vi "Main_v3.1.vi"() -> ()   [LabVIEW 2018]
doc: "Main VI for the controls"
uses:
  Components/PMCL Dynamic Signal Analyzer/Controls/DSA excitation specs.ctl
  Typedefs/StateDef_Enum.ctl
  <vilib>/Simulation/Scripting/Companion Diagram/SimConfigNode/SimParams.ctl
  <vilib>/Simulation/Scripting/Companion Diagram/SimConfigNode/_simSolvers.ctl
  <vilib>/Simulation/Implementation/Shared/SIMSCR Execution Mode.ctl
  <vilib>/Platform/TimedLoop/XDataNode/timing_clust.ctl
  <vilib>/Platform/TimedLoop/XDataNode/nitl_modes.ctl
  <vilib>/Platform/TimedLoop/XDataNode/wakeup.ctl
  <vilib>/Simulation/Param Hierarchy/Typedefs/SIMPH Param Control Actions.ctl
  <vilib>/Simulation/Implementation/Shared/SIM limit type.ctl
  <vilib>/Simulation/Scripting/Editor Utilities/SIM subVI tag data.ctl
  <vilib>/Simulation/Scripting/Editor Utilities/SIM subVI execution type.ctl
  <vilib>/Simulation/Implementation/Shared/NILVSim_ParamChanged.vi
  <vilib>/Simulation/Implementation/Shared/NILVSim_FinishedLate.vi
  <vilib>/Simulation/Implementation/Shared/NILVSIM_BeginStep.vi
  <vilib>/myRIO/Instrument Drivers/Onboard IO/AI/vis/Read.vi
  <vilib>/Simulation/Utility/Implementation/SIM SimulationParams.vi
  <vilib>/Simulation/ContinuousLinear/Implementation/NILVSim Integrator new.llb/SIM Integrator distributor (scalar).vi
  <vilib>/Simulation/Implementation/Shared/SIM Fire Discrete SubVI.vi
  <vilib>/Simulation/ContinuousLinear/Implementation/NILVSim Transfer Function Direct.llb/SIM Transfer Function Direct (SISO).vi
  <vilib>/Simulation/Utility/Implementation/SIM Halt.vi
  <vilib>/Simulation/SignalArithmetic/Implementation/NILVSim Gain.llb/SIM Gain (scalar).vi
  <vilib>/Simulation/ContinuousLinear/Implementation/NILVSim Integrator new.llb/SIM Integrator collector (scalar).vi
  <vilib>/Simulation/Implementation/Shared/NILVSim_Manager.vi
  <vilib>/Utility/error.llb/Clear Errors.vi
  <vilib>/Simulation/Implementation/Shared/NILVSim_FinalizeModel.vi
  <vilib>/Simulation/Utility/Implementation/NILVSim SimulationParams (core).vi
  <vilib>/Simulation/Implementation/Shared/SIM Fire Discrete SubVI (Core).vi
  <vilib>/myRIO/Common/Instrument Driver Framework/myRIO v1.0/AI/vis/myRIO v1.0 Close AI.vi
  <vilib>/myRIO/Common/Instrument Driver Framework/myRIO v1.0/AO/vis/myRIO v1.0 Close AO.vi
  <vilib>/myRIO/Common/Instrument Driver Framework/myRIO v1.0/AI/vis/myRIO v1.0 Unreserve AI.vi
  <vilib>/myRIO/Common/Instrument Driver Framework/myRIO v1.0/AO/vis/myRIO v1.0 Unreserve AO.vi
  <vilib>/myRIO/Common/Instrument Driver Framework/myRIO v1.0/Resource Manager/vis/myRIO v1.0 Unreserve Channel List.vi
  <vilib>/myRIO/Common/Instrument Driver Framework/myRIO v1.0/AI/vis/myRIO v1.0 Build MUX Configuration AI.vi
  <vilib>/myRIO/Common/Instrument Driver Framework/myRIO v1.0/AO/vis/myRIO v1.0 Build MUX Configuration AO.vi
  <vilib>/myRIO/Common/Instrument Driver Framework/myRIO v1.0/Resource Manager/vis/myRIO v1.0 Unreserve Channel.vi
  <vilib>/myRIO/Common/Instrument Driver Framework/myRIO v1.0/Resource Manager/vis/myRIO v1.0 Build Mutex Name.vi
  <vilib>/Simulation/Implementation/Shared/SIM Unbundle Sim Info.vi
  <vilib>/Simulation/Implementation/Shared/SIMSH Read Queue.vi
  <vilib>/Simulation/Implementation/Shared/NILVSim_Initialize.vi
  <vilib>/Utility/error.llb/Error Cluster From Error Code.vi
  <vilib>/myRIO/Common/Instrument Driver Framework/myRIO v1.0/AI/vis/myRIO v1.0 Read AI.vi
  <vilib>/myRIO/Common/Instrument Driver Framework/myRIO v1.0/AO/vis/myRIO v1.0 Write AO.vi
  <vilib>/Simulation/Utility/Implementation/NILVSim Get Time and IsAcceptedStep.vi
  <vilib>/Simulation/Implementation/Shared/NILVSim_GetModelError.vi
  <vilib>/Simulation/Implementation/Shared/SIM Bundle Sim Info.vi
  <vilib>/myRIO/Common/Instrument Driver Framework/Utilities/vis/Configuration Manager.vi
  <vilib>/myRIO/Common/Instrument Driver Framework/Utilities/vis/IO Manager.vi
  <vilib>/myRIO/Common/Instrument Driver Framework/myRIO v1.0/myRIO v1.0 Close.vi
  <vilib>/Simulation/Scripting/Companion Diagram/SimConfigNode/SimDog.xnode
  <vilib>/Platform/TimedLoop/XDataNode/XDataNode.xnode
  <vilib>/Simulation/Implementation/XNodeFramework/SimXNode/SimX.xnode
  Components/Timing/Timing.lvlib
  <vilib>/myRIO/Instrument Drivers/Onboard IO/AI/AI.lvlib
  <vilib>/myRIO/Instrument Drivers/Onboard IO/AO/AO.lvlib
  <vilib>/Platform/TimedLoop/XDataNode/XDNodeRunTimeDep.lvlib
  <vilib>/Analysis/NI_AALPro.lvlib
  <vilib>/ptbypt/NI_PtbyPt.lvlib
  <vilib>/Simulation/ContinuousLinear/Implementation/NILVSim Integrator new.llb/SIM Integrator (scalar).vi
  <vilib>/Simulation/Implementation/Shared/NI_SIM_Implementation.lvlib
panel:
  in  "System Stop Button":bool
  in  "Pause chart?":bool
  in  "Controller Params":enum32{"Page 1"}(tab)
  in  "Kp":dbl=1.0 min=0.0
  in  "Controller On?":bool
  out "Status":string
  in  "Ref. Gen.":enum32{"Analog In", "Manual", "Wave Gen", "DSA"}(tab)=enum."Manual"
  in  "Ref. cmd.":dbl(slide) step=1.0 scale=-10.0..10.0 scale format="%#.1f"
  in  "Signal Cluster":T1={"phase"=0.0, "amplitude"=1.0, "frequency"=1.0, "offset"=1.0, "Signal"=enum."Square"} {"offset" format="%0.2f"; "frequency" format="%0.2f"; "amplitude" format="%0.2f"; "phase" format="%0.2f"}
  out "DSA \nRunning?":bool
  in  "Stop DSA":bool
  in  "Start DSA":bool
  in  "DSA excitation specs":T2={"Initial Freq. [Hz]"=10.0, "Final Freq. [Hz]"=999.0, "# pts. in interval"=50, "Samping Time [s]"=0.001, "Amplitude [V]"=10.0, "Offset [V]"=0.0, "Freq Units (F: rad/s, T: Hz)"=TRUE}
  in  "Loop Timing":enum32{"CD&Sim", "Ref. gen", "UI"}(tab)
  out "# Finished\nLate counter":dbl
  in  "CD&Sim\nLoop Rate (Hz)":dbl=2000.0 format="%#_4p"
  out "# Finished\nLate counter":dbl
  in  "Ref. Gen.\nLoop Rate (Hz)":dbl=2000.0 format="%#_4p"
  in  "UI Loop rate (Hz)":dbl=1000.0 format="%#_6p"
  in  "Display Waveforms":enum32{"Controller Signals", "DSA "}(tab)
  out "Control Effort":dbl(graph)
  out "Waveform Chart":cluster{"Double":dbl, "Numeric":dbl}(graph)
  out "Phase Bode Plot":cluster{dbl[], dbl[]}(graph)
  out "Magnitude Bode Plot":cluster{dbl[], dbl[]}(graph)
  out "DSA Signals":cluster{"Double":dbl, "Double":dbl}(graph)
  # "Connect the Reference Signal \nto C/AI 1 of the myRIO."
  # "Pinout Config.:\nPort C/AI0 : Plant output being read by the myRIO\nPort C/AI1 : Reference signal for the control loop\nPort C/AO0 : Control effort signal to the plant"
  # "Ensure the excitation specs, cycle specs and\nCH0, CH1 inputs to the droppable DSA in the\nDSA loop are correctly set before starting DSA."
  # "Control Loop Timing"
  # "Ref.  Gen. Loop Timing"
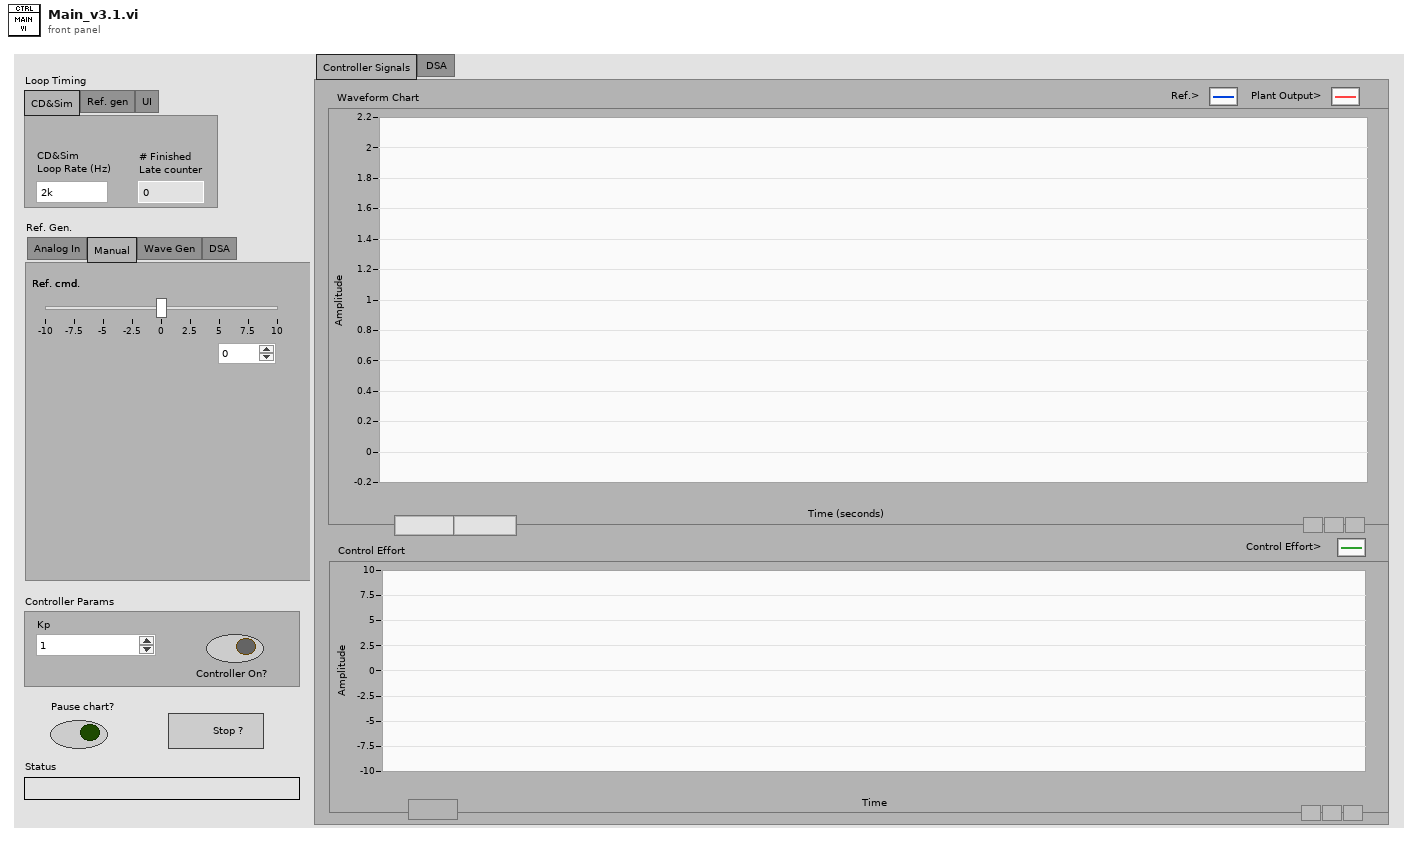
[diagram p1: front panel]
types:
  T1 = cluster{"phase":dbl, "amplitude":dbl, "frequency":dbl, "offset":dbl, "Signal":enum16{"Sine", "Square", "Sawtooth"}}
  T2 = typedef "DSA excitation specs.ctl" = cluster{"Initial Freq. [Hz]":dbl, "Final Freq. [Hz]":dbl, "# pts. in interval":i16, "Samping Time [s]":dbl, "Amplitude [V]":dbl, "Offset [V]":dbl, "Freq Units (F: rad/s, T: Hz)":bool}
  T3 = typedef "StateDef_Enum.ctl" = enum16{"Initialize", "Wait", "Shutdown"}
  T4 = typedef "XDNodeRunTimeDep.lvlib/timing_clust.ctl" = cluster{"Expected End [f-1]":u64, "Actual End [f-1]":u64, "Finished Late? [f-1]":bool, "Expected End [i-1]":u64, "Actual End [i-1]":u64, "Finished Late? [i-1]":bool, "Expected Start [i]":u64, "Actual Start [i]":u64, "Expected Start [f]":u64, "Actual Start [f]":u64, "Source Name":string, "Structure Name":string, "Period":i64, "Deadline":i64, "Offset":i64, "Start":i64, "Priority":i32, "Timeout":i32, "Mode":T5, "Wakeup Reason":T6, "Error":errorcluster, "Source Type":string, "Secondary Source Type":string, "Global End Time":u64, "Global Start Time":u64, "Frame Duration":u64, "Iteration Duration":u64, "Assigned CPU":i32, "I/O Scan Engine Mode":u32}
  T5 = typedef "XDNodeRunTimeDep.lvlib/nitl_modes.ctl" = enum32{"No Change", "Process missed periods, maintain original phase", "Discard missed periods, maintain original phase", "Process missed periods, ignore original phase", "Discard missed periods, ignore original phase"}
  T6 = typedef "XDNodeRunTimeDep.lvlib/wakeup.ctl" = enum32{"Normal", "Aborted", "Asynchronous wakeup", "Timing source error", "Timed loop error", "Timeout"}
  T7 = typedef "AI.lvlib/AI Reference.ctl" = cluster{"myRIO Reference":T8, "AI Channels List":T12, "AI Scaling Constants List":T14}
  T8 = typedef "myRIO Generic Hardware Reference.ctl" = cluster{"myRIO Model":T9, "myRIO Hardware Reference":T10}
  T9 = typedef "Hardware Version Enum.ctl" = enum16{"Unknown", "myRIO-1900", "myRIO-1950", "roboRIO", "NI ELVIS RIO CM", "ELVIS III"}
  T10 = typedef "myRIO v1.0 Reference.ctl" = cluster{"Generic FPGA Reference":T11, "Allow multiple opens":bool}
  T11 = typedef "Generic FPGA Reference.ctl" = refnum<k20>
  T12 = typedef "AI Channels List.ctl" = T13[]
  T13 = typedef "AI Channels Enum.ctl" = enum16{"Not Connected", "AudioIn/Left", "AudioIn/Right", "C/AI0", "C/AI1", "A/AI0", "A/AI1", "A/AI2", "A/AI3", "A/AI4", "A/AI5", "A/AI6", "A/AI7", "B/AI0", "B/AI1", "B/AI2", "B/AI3", "B/AI4", "B/AI5", "B/AI6", "B/AI7", "AI/AI0", "AI/AI1", "AI/AI2", "AI/AI3", "A/AI0 (DIFF)", "A/AI1 (DIFF)", "A/AI2 (DIFF)", "A/AI3 (DIFF)", "B/AI0 (DIFF)", "B/AI1 (DIFF)", "B/AI2 (DIFF)", "B/AI3 (DIFF)"}
  T14 = typedef "Analog Scaling Constants List.ctl" = T15[]
  T15 = typedef "Analog Scaling Constants.ctl" = cluster{"LSB Weight (Volts)":dbl, "Offset (Volts)":dbl, "Signed?":bool}
  T16 = typedef "AO.lvlib/AO Reference.ctl" = cluster{"myRIO Reference":T8, "AO Channel List":T17, "AO Scaling Constant List":T14}
  T17 = typedef "AO Channels List.ctl" = T18[]
  T18 = typedef "AO Channels Enum.ctl" = enum16{"Not Connected", "AudioOut/Left", "AudioOut/Right", "C/AO0", "C/AO1", "A/AO0", "A/AO1", "B/AO0", "B/AO1"}
  T19 = cluster{"Cycles To Settle (M)":i16, "Cycles To Calculate (N)":i16}
  T20 = cluster{"Analog In CH1":dbl, "Analog In CH0":dbl}
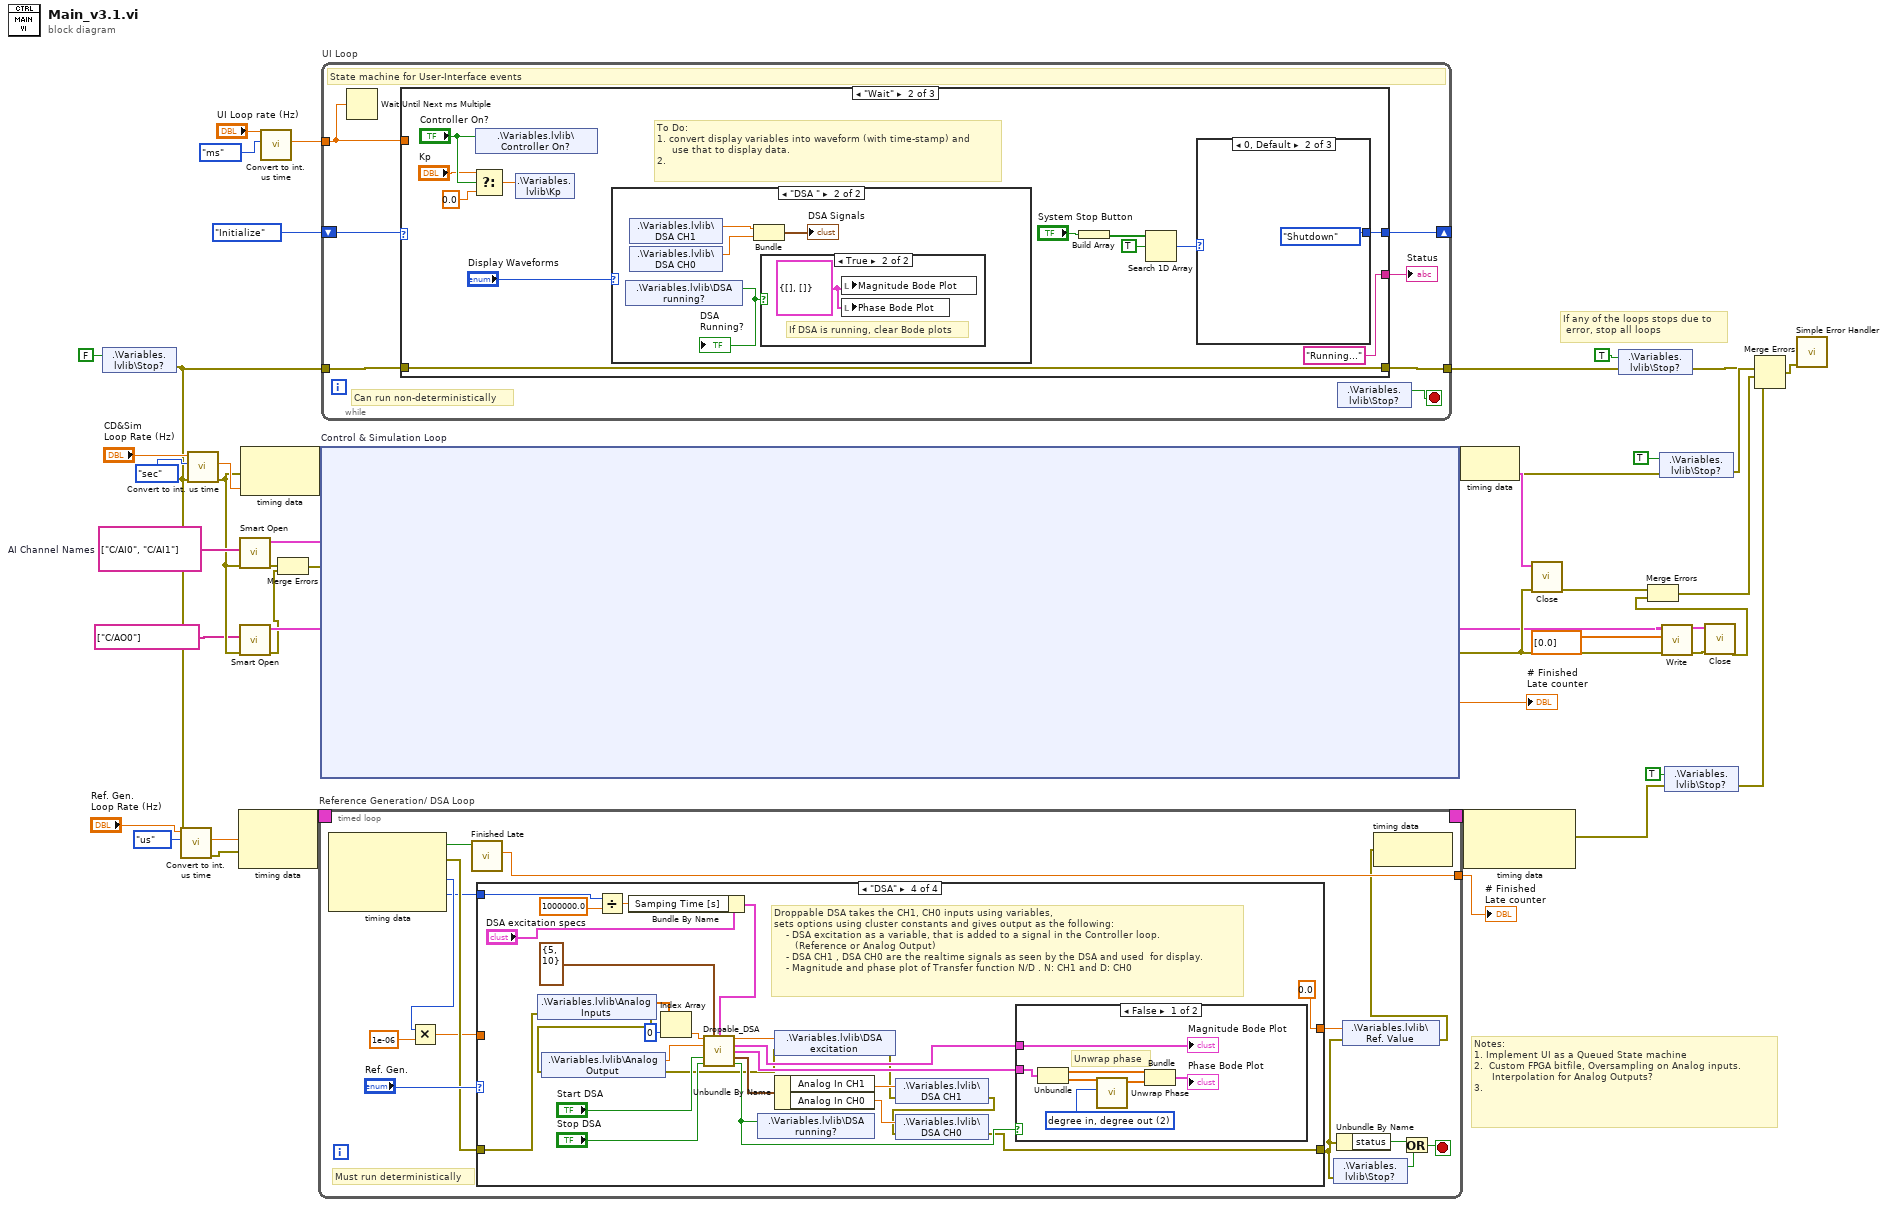
[diagram p0: block diagram]
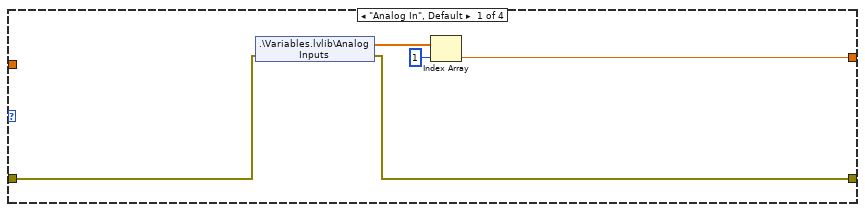
[diagram p2: hidden frame]
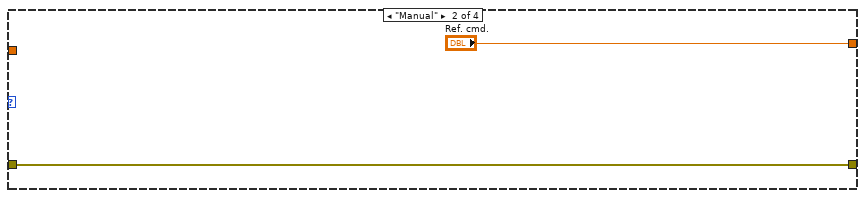
[diagram p3: hidden frame]
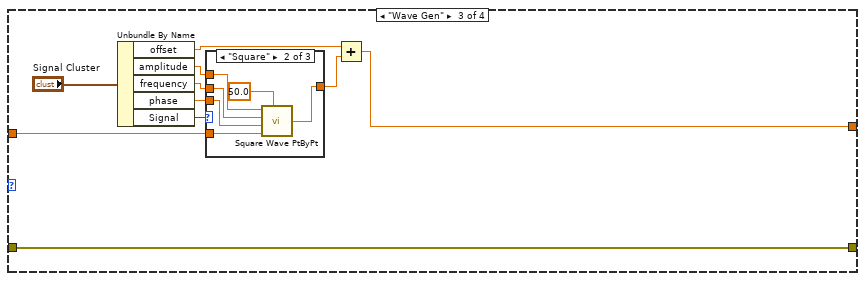
[diagram p4: hidden frame]
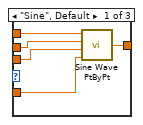
[diagram p5: hidden frame]
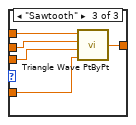
[diagram p6: hidden frame]
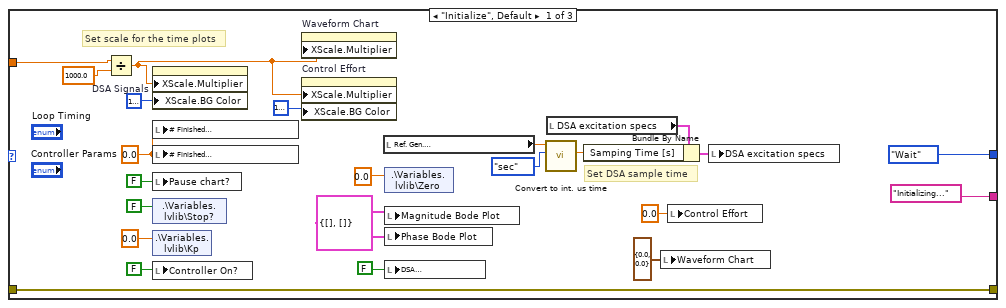
[diagram p8: hidden frame]
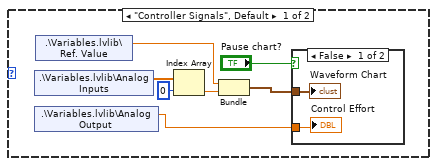
[diagram p9: hidden frame]
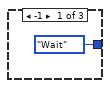
[diagram p12: hidden frame]
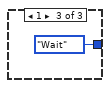
[diagram p13: hidden frame]
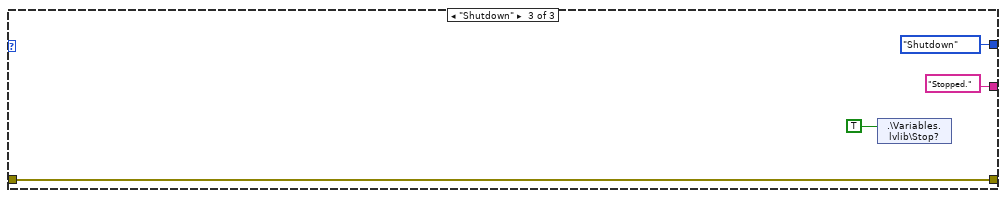
[diagram p14: hidden frame]
diagram:
  w36 = tag[] ["C/AI0", "C/AI1"]  # AI Channel Names
  # "Notes:\n1. Implement UI as a Queued State machine\n2.  Custom FPGA bitfile, Oversampling on Analog inputs. \n      Interpolation for Analog Outputs?\n3."
  # "If any of the loops stops due to\n error, stop all loops"
  n1 = shared-variable ".\\Variables.lvlib\\Stop?"(FALSE ("Stop?")) -> (error out=w1:errorcluster)  [unwired: 1 in]
  n2 = call "Convert to int. us time.vi"("error in (no error)"=w1, "Int. Time Unit"=enum16{"sec", "us", "ms"}."us", "Sample rate (Hz)"="Ref. Gen.\nLoop Rate (Hz)") -> ("error out"=w21:errorcluster, "Int.  time [unit]"=w25:dbl)  [unwired: 6 in, 1 out]
  n3 = call "Convert to int. us time.vi"("error in (no error)"=w1, "Int. Time Unit"=enum16{"sec", "us", "ms"}."sec", "Sample rate (Hz)"="CD&Sim\nLoop Rate (Hz)") -> ("error out"=w22:errorcluster, "Int.  time [unit]"=w41:dbl)  [unwired: 6 in, 1 out]
  n4 = node-c288(w25, w21) -> (w28:T4)
  n5 = call <vilib>:"Smart Open.vi"("error in (no error)"=w22, "Channel Names"=w36) -> ("error out"=w37:errorcluster, "AI Ref Out"=w38:T7)  [unwired: 8 in]
  n6 = call <vilib>:"Smart Open.vi"("error in (no error)"=w22, "Channel Names"=tag[] ["C/AO0"]) -> ("error out"=w33:errorcluster, "AO Ref Out"=w35:T16)  [unwired: 8 in]
  n7 = node-c288(w22, w41) -> (w45:variant)
  n8 = call "Convert to int. us time.vi"("Int. Time Unit"=enum16{"sec", "us", "ms"}."ms", "Sample rate (Hz)"="UI Loop rate (Hz)") -> ("Int.  time [unit]"=w6:dbl)  [unwired: 7 in, 2 out]
  n9 = Merge Errors(w37, w33) -> (w34:errorcluster)
  n10 = timed-loop "Reference Generation/ DSA Loop" {
    timing: w28 -> [_]
    timing-out: [_] -> w27
    tunnel: [w59] -> w23
    stop <- w53 stop-if-true
    # "Must run deterministically"
    n11 = node-c288() -> (w60:bool, w56:errorcluster, w50:i64, w49:i64)  [unwired: 1 in]
    n12 = Multiply(x=w50, y=1e-06) -> (x*y=w52:dbl)
    n13 = call "Finished Late.vi"("Finished \nLate?"=w60) -> ("# Finished\nLate counter"=w59:dbl)  [unwired: 8 in, 2 out]
    n14 = case shown="\"DSA\"" "Ref. Gen." {
      tunnel: [w65 "Ref. cmd." w70 0.0 ("Ref. cmd.")] -> w57
      tunnel: w56 -> [w63 w66 w69 w98]
      tunnel: [w62 w66 w69 w95] -> w47
      tunnel: w52 -> [_ _ w68 _]
      tunnel: w49 -> [_ _ _ w105]
      frame "Analog In", Default {
        n15 = shared-variable ".\\Variables.lvlib\\Analog Inputs"(error in=w63) -> (w64:dbl[], error out=w62:errorcluster)
        n16 = Index Array(array=w64, index=1) -> (element=w65:dbl)
      }
      frame "Manual" {
      }
      frame "Wave Gen" {
        n17 = Unbundle By Name("Signal Cluster") -> ("offset"=w71:dbl, "amplitude"=w74:dbl, "frequency"=w73:dbl, "phase"=w72:dbl, "Signal"=w75:enum16{"Sine", "Square", "Sawtooth"})
        n18 = case shown="\"Square\"" w75 {
          tunnel: [w82 w87 w93] -> w77
          tunnel: w74 -> [w81 w86 w92]
          tunnel: w73 -> [w80 w85 w91]
          tunnel: w72 -> [w79 w84 w90]
          tunnel: w68 -> [w78 w83 w89]
          frame "Sine", Default {
            n19 = call <vilib>:"Sine Wave PtByPt.vi"("time"=w78, "phase"=w79, "frequency"=w80, "amplitude"=w81) -> ("sine wave"=w82:dbl)
          }
          frame "Square" {
            n20 = call <vilib>:"Square Wave PtByPt.vi"("amplitude"=w86, "frequency"=w85, "phase"=w84, "time"=w83, "duty cycle (%)"=50.0) -> ("square wave"=w87:dbl)
          }
          frame "Sawtooth" {
            n21 = call <vilib>:"Triangle Wave PtByPt.vi"("time"=w89, "phase"=w90, "frequency"=w91, "amplitude"=w92) -> ("triangle wave"=w93:dbl)
          }
        }
        n22 = Add(x=w71, y=w77) -> (x+y=w70:dbl)
      }
      frame "DSA" {
        # "Droppable DSA takes the CH1, CH0 inputs using variables, \nsets options using cluster constants and gives output as the following:\n    - DSA excitation as a variable, that is added to a signal in the Controller loop. \n       (Reference or Analog Output)\n    - DSA CH1 , DSA CH0 are the realtime signals as seen by the DSA and used  for display.\n    - Magnitude and phase plot of Transfer function N/D . N: CH1 and D: CH0"
        n23 = shared-variable ".\\Variables.lvlib\\Analog Inputs"(error in=w98) -> (w111:dbl[], error out=w100:errorcluster)
        n24 = shared-variable ".\\Variables.lvlib\\Analog Output"(error in=w100) -> (w108:dbl, error out=w99:errorcluster)
        n25 = Divide(x=w105, y=1000000.0) -> (x/y=w103:dbl)
        n26 = Bundle By Name(cluster="DSA excitation specs", "Samping Time [s]"=w103) -> (w102:T2)
        n27 = Index Array(array=w111, index=0) -> (element=w109:dbl)
        n28 = call "Dropable_DSA.vi"("Analog In CH1"=w109, "Cycle Specs"=T19 {"Cycles To Settle (M)"=5, "Cycles To Calculate (N)"=10}, "Excitation Specs"=w102, "Analog In CH0"=w108, "START"="Start DSA", "STOP"="Stop DSA") -> ("Analog Out"=w117:dbl, "Bode Magnitude"=w107:cluster{dbl[], dbl[]}, "Bode Phase"=w106:cluster{dbl[], dbl[]}, "Live signals"=w114:T20, "Running"=w101:bool)  [unwired: 4 in, 1 out]
        n29 = shared-variable ".\\Variables.lvlib\\DSA running?"(w101) -> ()  [unwired: 1 in, 1 out]
        n30 = shared-variable ".\\Variables.lvlib\\DSA excitation"(w117, error in=w99) -> (error out=w97:errorcluster)
        n31 = Unbundle By Name(w114) -> ("Analog In CH1"=w113:dbl, "Analog In CH0"=w112:dbl)
        n32 = shared-variable ".\\Variables.lvlib\\DSA CH1"(w113, error in=w97) -> (error out=w96:errorcluster)
        n33 = shared-variable ".\\Variables.lvlib\\DSA CH0"(w112, error in=w96) -> (error out=w95:errorcluster)
        n34 = case shown="False" w101 {
          tunnel: w107 -> [w120 _]
          tunnel: w106 -> [w122 _]
          frame False {
            w124 = 2 items=["radian in, radian out", "radian in, degree out", "degree in, degree out", "degree in, radian out"] ("phase unit")
            # "Unwrap phase"
            n35 = Unbundle(w122) -> (w126:dbl[], w123:dbl[])
            n36 = call <vilib>:"Unwrap Phase.vi"("phase unit"=w124, "Phase"=w123) -> ("Unwrapped Phase"=w125:dbl[])  [unwired: 8 in, 1 out]
            n37 = Bundle(w126, "Unwrapped Phase"=w125) -> (→"Phase Bode Plot":cluster{dbl[], "Unwrapped Phase":dbl[]})  [unwired: 1 in]
            "Magnitude Bode Plot" <- w120
          }
          frame True {
          }
        }
      }
    }
    n38 = shared-variable ".\\Variables.lvlib\\Stop?"(error in=w47) -> (w54:bool)  [unwired: 1 out]
    n39 = Unbundle By Name(w47) -> ("status"=w55:bool)
    n40 = shared-variable ".\\Variables.lvlib\\Ref. Value"(w57, error in=w47) -> (error out=w48:errorcluster)
    n41 = node-c288(w48) -> ()  [unwired: 1 out]
    n42 = Or(x=w55, y=w54) -> (x .or. y?=w53:bool)
  }
  "# Finished\nLate counter" <- w23
  n43 = node-c254 "Control & Simulation Loop"(w45, w38, w34, w35) -> (w44:variant, →"# Finished\nLate counter":dbl, w11:T16, w14:errorcluster, w32:T7)
  n44 = while "UI Loop" {
    shift-right: [w140] -> _
    shift-left: StateDef_Enum."Initialize" ("State defining Enum") -> [w141]
    tunnel: w1 -> [w139]
    tunnel: [w138] -> w5
    tunnel: w6 -> [w135]
    stop <- w136 stop-if-true
    # "Can run non-deterministically"
    # "State machine for User-Interface events"
    n45 = Wait Until Next ms Multiple(millisecond multiple=w135) -> ()  [unwired: 1 out]
    n46 = case shown="\"Wait\"" w141 {
      tunnel: [StateDef_Enum."Wait" ("State defining Enum") w173 StateDef_Enum."Shutdown" ("State defining Enum")] -> w140
      tunnel: w139 -> [w161 w171 w197]
      tunnel: [w161 w171 w197] -> w138
      tunnel: ["Initializing..." ("Status") "Running..." ("Status") "Stopped." ("Status")] -> w137
      tunnel: w135 -> [w159 _ _]
      frame "Initialize", Default {
        w153 = cluster{dbl[], dbl[]} {[], []} ("Magnitude Bode Plot")
        w155 = 0.0 ("# Finished\nLate counter")
        # "Set DSA sample time"
        # "Set scale for the time plots"
        n47 = Divide(x=w159, y=1000.0) -> (x/y=w145:dbl)
        n48 = property on="DSA Signals" class="WFChart (strict)"("XScale.Multiplier"=w145, "XScale.BG Color"=u32 16777216) -> ()  [unwired: 2 in, 2 out]
        n49 = local write "# Finished\nLate counter"(w155) -> ()
        n50 = local write "# Finished\nLate counter"(w155) -> ()
        n51 = local write "Pause chart?"(FALSE ("Pause chart?")) -> ()
        n52 = shared-variable ".\\Variables.lvlib\\Stop?"(FALSE ("Stop?")) -> ()  [unwired: 1 in, 1 out]
        n53 = shared-variable ".\\Variables.lvlib\\Kp"(0.0 ("Kp")) -> ()  [unwired: 1 in, 1 out]
        n54 = local write "Controller On?"(FALSE ("Controller On?")) -> ()
        n55 = property on="Waveform Chart" class="WFChart (strict)"("XScale.Multiplier"=w145) -> ()  [unwired: 2 in, 2 out]
        n56 = property on="Control Effort" class="WFChart (strict)"("XScale.Multiplier"=w145, "XScale.BG Color"=u32 16777216) -> ()  [unwired: 2 in, 2 out]
        n57 = local read "Ref. Gen.\nLoop Rate (Hz)"() -> (w148:dbl)
        n58 = shared-variable ".\\Variables.lvlib\\Zero"(0.0 ("Zero")) -> ()  [unwired: 1 in, 1 out]
        n59 = local write "Magnitude Bode Plot"(w153) -> ()
        n60 = local write "Phase Bode Plot"(w153) -> ()
        n61 = local write "DSA \nRunning?"(FALSE ("DSA \nRunning?")) -> ()
        n62 = call "Convert to int. us time.vi"("Int. Time Unit"=enum16{"sec", "us", "ms"}."sec", "Sample rate (Hz)"=w148) -> ("Int.  time [unit]"=w146:dbl)  [unwired: 7 in, 2 out]
        n63 = local read "DSA excitation specs"() -> (w150:T2)
        n64 = Bundle By Name(cluster=w150, "Samping Time [s]"=w146) -> (w149:T2)
        n65 = local write "Waveform Chart"(cluster{"Double":dbl, "Numeric":dbl} {"Double"=0.0, "Numeric"=0.0} ("Waveform Chart")) -> ()
        n66 = local write "Control Effort"(0.0 ("Control Effort")) -> ()
        n67 = local write "DSA excitation specs"(w149) -> ()
      }
      frame "Wait" {
        # "To Do:\n1. convert display variables into waveform (with time-stamp) and\n     use that to display data.\n2."
        n68 = Select(t="Kp", s="Controller On?", f=0.0) -> (s? t:f=w169:dbl)
        n69 = shared-variable ".\\Variables.lvlib\\Controller On?"("Controller On?") -> ()  [unwired: 1 in, 1 out]
        n70 = shared-variable ".\\Variables.lvlib\\Kp"(w169) -> ()  [unwired: 1 in, 1 out]
        n71 = case shown="\"DSA \"" "Display Waveforms" {
          frame "Controller Signals", Default {
            n72 = shared-variable ".\\Variables.lvlib\\Analog Inputs"() -> (w183:dbl[])  [unwired: 1 in, 1 out]
            n73 = shared-variable ".\\Variables.lvlib\\Analog Output"() -> (w177:dbl)  [unwired: 1 in, 1 out]
            n74 = shared-variable ".\\Variables.lvlib\\Ref. Value"() -> (w180:dbl)  [unwired: 1 in, 1 out]
            n75 = Index Array(array=w183, index=0) -> (element=w182:dbl)
            n76 = Bundle("Double"=w180, "Numeric"=w182) -> (w178:cluster{"Double":dbl, "Numeric":dbl})  [unwired: 1 in]
            n77 = case shown="False" "Pause chart?" {
              tunnel: w178 -> [w185 _]
              tunnel: w177 -> [w184 _]
              frame False {
                "Waveform Chart" <- w185
                "Control Effort" <- w184
              }
              frame True {
              }
            }
          }
          frame "DSA " {
            n78 = shared-variable ".\\Variables.lvlib\\DSA running?"() -> (w186:bool)  [unwired: 1 in, 1 out]
            "DSA \nRunning?" <- w186
            n79 = shared-variable ".\\Variables.lvlib\\DSA CH1"() -> (w188:dbl)  [unwired: 1 in, 1 out]
            n80 = shared-variable ".\\Variables.lvlib\\DSA CH0"() -> (w187:dbl)  [unwired: 1 in, 1 out]
            n81 = Bundle("Double"=w188, "Double"=w187) -> (→"DSA Signals":cluster{"Double":dbl, "Double":dbl})  [unwired: 1 in]
            n82 = case shown="True" w186 {
              frame False {
              }
              frame True {
                w190 = cluster{dbl[], dbl[]} {[], []} ("Magnitude Bode Plot")
                # "If DSA is running, clear Bode plots"
                n83 = local write "Magnitude Bode Plot"(w190) -> ()
                n84 = local write "Phase Bode Plot"(w190) -> ()
              }
            }
          }
        }
        n85 = Build Array("System Stop Button") -> (w175:bool[])
        n86 = Search 1D Array(1D array=w175, element=TRUE) -> (index of element=w172:i32)  [unwired: 1 in]
        n87 = case shown="0, Default" w172 {
          tunnel: [StateDef_Enum."Wait" ("State defining Enum") StateDef_Enum."Shutdown" ("State defining Enum") StateDef_Enum."Wait" ("State defining Enum")] -> w173
          frame -1 {
          }
          frame 0, Default {
          }
          frame 1 {
          }
        }
      }
      frame "Shutdown" {
        n88 = shared-variable ".\\Variables.lvlib\\Stop?"(TRUE) -> ()  [unwired: 1 in, 1 out]
      }
    }
    "Status" <- w137
    n89 = shared-variable ".\\Variables.lvlib\\Stop?"() -> (w136:bool)  [unwired: 1 in, 1 out]
  }
  n90 = node-c288(w44) -> (w20:errorcluster)
  n91 = node-c288(w27) -> (w17:errorcluster)  [unwired: 1 out]
  n92 = call <vilib>:"Close.vi"("error in (no error)"=w14, "AI Ref In"=w32) -> ("error out"=w31:errorcluster)  [unwired: 9 in]
  n93 = shared-variable ".\\Variables.lvlib\\Stop?"(TRUE ("Stop?"), error in=w5) -> (error out=w4:errorcluster)
  n94 = shared-variable ".\\Variables.lvlib\\Stop?"(TRUE ("Stop?"), error in=w20) -> (error out=w19:errorcluster)
  n95 = call <vilib>:"Write.vi"("error in (no error)"=w14, "Values"=dbl[] [0.0], "AO Ref In"=w11) -> ("error out"=w13:errorcluster, "AO Ref Out"=w12:T16)  [unwired: 6 in]
  n96 = shared-variable ".\\Variables.lvlib\\Stop?"(TRUE ("Stop?"), error in=w17) -> (error out=w16:errorcluster)
  n97 = call <vilib>:"Close.vi"("error in (no error)"=w13, "AO Ref In"=w12) -> ("error out"=w30:errorcluster)  [unwired: 9 in]
  n98 = Merge Errors(w31, w30) -> (w29:errorcluster)
  n99 = Merge Errors(w4, w19, w29, w16) -> (w39:errorcluster)
  n100 = call <vilib>:"Simple Error Handler.vi"("error in (no error)"=w39) -> ()  [unwired: 4 in, 5 out]
